vi "settings_options_general.vi"(8 "error in (no error)":errorcluster, 11 "Selection Done?":bool) -> (0 "error IO":errorcluster, 3 "button pressed":T1(ring))   [LabVIEW 2019, in "ZenGage v3.0 UI.lvclass"]
uses:
  ZenGage v3.0 UI.lvclass
panel:
  in  "Exit":bool
  out "Dialog Box out":string=" CHOOSE AN ACTION"
  in  "Diagnostics":bool
  in  "Edit limits":bool
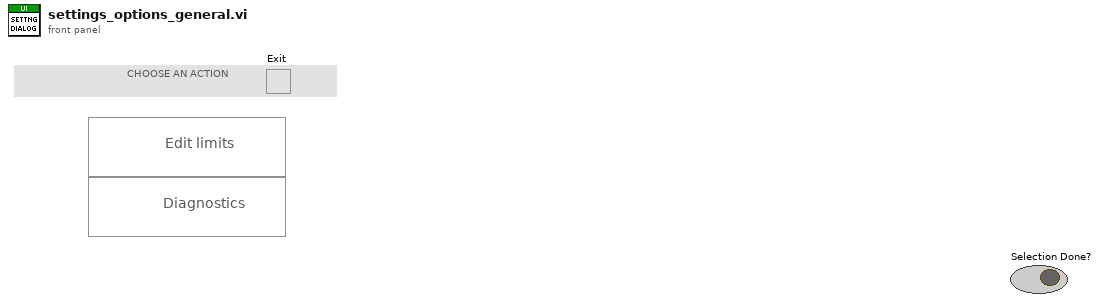
[diagram p1: front panel]
types:
  T1 = enum16{"cancel", "edit tolerance", "diagnostics"}
  T2 = enum8{"Enabled", "Disabled", "Disabled and Grayed Out"}
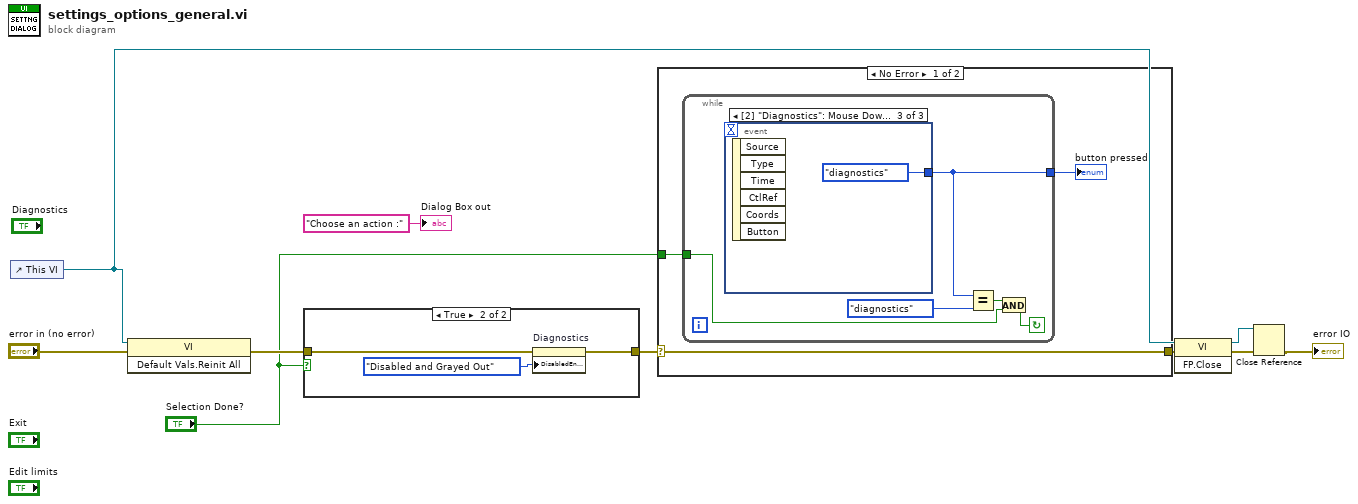
[diagram p0: block diagram]
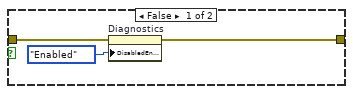
[diagram p2: hidden frame]
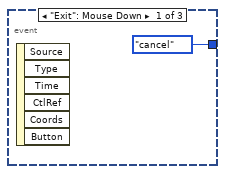
[diagram p3: hidden frame]
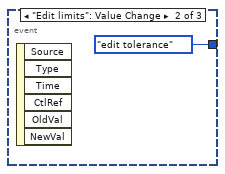
[diagram p4: hidden frame]
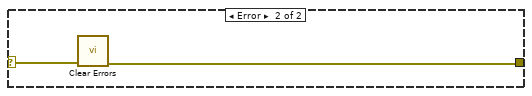
[diagram p5: hidden frame]
diagram:
  n1 = control-ref of="This VI"() -> (w5:refnum<vi>)
  n2 = invoke class="VI" method="Default Vals.Reinit All"(reference=w5, error in="error in (no error)") -> (error out=w7:errorcluster)  [unwired: 1 in, 2 out]
  n3 = case shown="True" "Selection Done?" {
    tunnel: w7 -> [w12 w16]
    tunnel: [w11 w15] -> w6
    frame False {
      n4 = property on="Diagnostics" class="Bool (strict)"(error in=w12, "DisabledEnum"=T2."Enabled" ("Disabled")) -> (error out=w11:errorcluster)  [unwired: 1 in, 1 out]
    }
    frame True {
      n5 = property on="Diagnostics" class="Bool (strict)"(error in=w16, "DisabledEnum"=T2."Disabled and Grayed Out" ("Disabled")) -> (error out=w15:errorcluster)  [unwired: 1 in, 1 out]
    }
  }
  n6 = case shown="No Error" w6 {
    selector: w6 -> [w18 w29]
    tunnel: [w18 w28] -> w10
    tunnel: "Selection Done?" -> [w17 _]
    frame No Error {
      n7 = while {
        tunnel: [w24] -> w19
        tunnel: w17 -> [w21]
        stop <- w20 continue-if-true
        n8 = event shown="[2] \"Diagnostics\": Mouse Down" {
          selector: _ -> [_ _ _]
          dyn-events: _ -> [_ _ _]
          timeout: _ -> [_ _ _]
          tunnel: [T1."cancel" T1."edit tolerance" T1."diagnostics"] -> w24
          event "Exit": Mouse Down {
            n9 = event-data() -> ()  [unwired: 1 in, 6 out]
          }
          event "Edit limits": Value Change {
            n10 = event-data() -> ()  [unwired: 1 in, 6 out]
          }
          event "Diagnostics": Mouse Down {
            n11 = event-data() -> ()  [unwired: 1 in, 6 out]
          }
        }
        n12 = Equal?(x=w24, y=T1."diagnostics") -> (x = y?=w22:bool)
        n13 = And(x=w22, y=w21) -> (x .and. y?=w20:bool)
      }
      "button pressed" <- w19
    }
    frame Error {
      n14 = call <vilib>:"Clear Errors.vi"("error in (no error)"=w29) -> ("error out"=w28:errorcluster)  [unwired: 5 in, 1 out]
    }
  }
  n15 = invoke class="VI" method="FP.Close"(reference=w5, error in=w10) -> (reference out=w3:refnum<vi>, error out=w4:errorcluster)  [unwired: 1 in, 1 out]
  n16 = Close Reference(reference=w3, error in (no error)=w4) -> (error out=→"error IO":errorcluster)
  "Dialog Box out" <- "Choose an action :" ("String")
